vi "Parse Global Header.vi"(8 "error in":errorcluster, 10 "Bytes in":u8[](array[numeric]), 11 "pcap Parse and Build in":refnum<class "pcap_Parse_Build_CIF.lvclass">) -> (0 "error out":errorcluster, 1 "Global Header":T1 {"magic number" format="%.0x"}, 2 "Bytes out":u8[](array[numeric]), 3 "pcap Parse and Build out":refnum<class "pcap_Parse_Build_CIF.lvclass">)   [LabVIEW 2021, in "pcap_Parse_Build_CIF.lvclass"]
uses:
  pcap_Parse_Build_CIF.lvclass
  Typedef/Global Header.ctl
  Typedef/Errors.ctl
  Typedef/Time Format.ctl
  Typedef/File Format.ctl
  <vilib>/CIF Foundation/CIF Utilities/DataTypes/Typedef/Endian.ctl
  pcap_Parse_Build_CIF.lvclass/pcap_Parse_Build_CIF.ctl
  Utilities/Add Error Core.vi
  <vilib>/CIF Foundation/CIF Utilities/DataTypes/DataTypes_CIF_U.lvlib
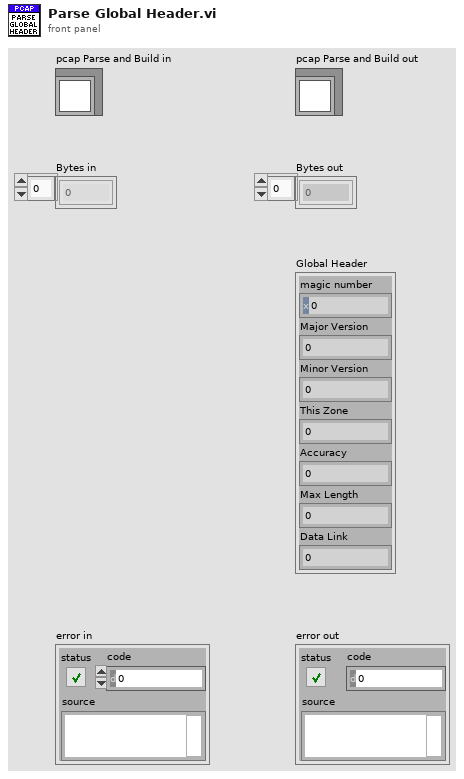
[diagram p1: front panel]
types:
  T1 = typedef "pcap_Parse_Build_CIF.lvclass/Global Header.ctl" = cluster{"magic number":u32, "Major Version":u16, "Minor Version":u16, "This Zone":u32, "Accuracy":u32, "Max Length":u32, "Data Link":u32}
  T2 = typedef "pcap_Parse_Build_CIF.lvclass/Errors.ctl" = enum16{"Invalid Global Header", "Out of Data"}
  T3 = typedef "pcap_Parse_Build_CIF.lvclass/Time Format.ctl" = enum16{"us", "ns"}
  T4 = typedef "pcap_Parse_Build_CIF.lvclass/File Format.ctl" = cluster{"Endian":T5, "Time Format":T3}
  T5 = typedef "DataTypes_CIF_U.lvlib/Endian.ctl" = enum16{"Little Endian", "Big Endian"}
  T6 = enum16{"big-endian, network order", "native, host order", "little-endian"}[]
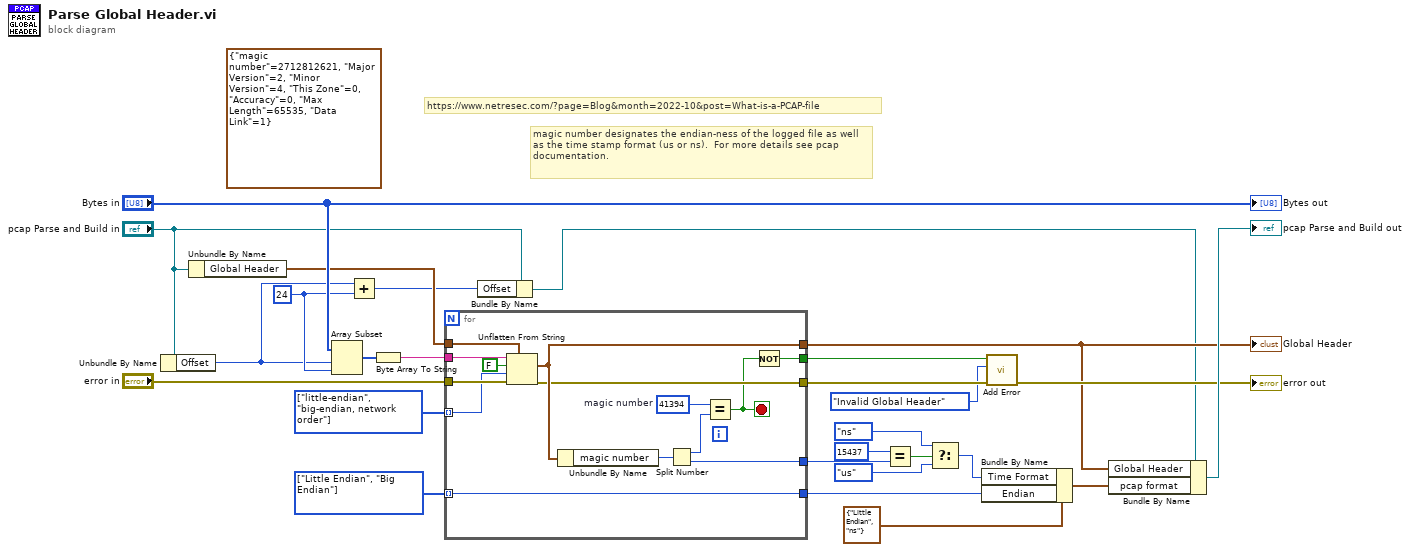
[diagram p0: block diagram]
diagram:
  w16 = T5[] [enum."Little Endian", enum."Big Endian"] items=["Little Endian", "Big Endian"]
  w18 = 24 ("y")
  (unwired) T1 {"magic number"=2712812621, "Major Version"=2, "Minor Version"=4, "This Zone"=0, "Accuracy"=0, "Max Length"=65535, "Data Link"=1} ("Global Header")
  w26 = T6 [enum."little-endian", enum."big-endian, network order"] items=["big-endian, network order", "native, host order", "little-endian"]
  # "https://www.netresec.com/?page=Blog&month=2022-10&post=What-is-a-PCAP-file"
  # "magic number designates the endian-ness of the logged file as well as the time stamp format (us or ns).  For more details see pcap documentation."
  n1 = Unbundle By Name("pcap Parse and Build in") -> ("Offset"=w4:i32)
  n2 = Unbundle By Name("pcap Parse and Build in") -> ("Global Header"=w5:T1)
  n3 = Array Subset(array="Bytes in", index=w4, length=w18) -> (w17:u8[])
  n4 = Add(x=w4, y=w18) -> (x+y=w2:i32)
  n5 = Byte Array To String(unsigned byte array=w17) -> (string=w27:string)
  n6 = for {
    tunnel: w27 -> [w41]
    tunnel: w26 -> [w30] mode=indexing
    tunnel: [w39] -> w6
    tunnel: [w31] -> w21
    tunnel: [w29] -> w8
    tunnel: [w35] -> w25
    tunnel: [w34] -> w10
    tunnel: "error in" -> [w33]
    tunnel: w16 -> [w31] mode=indexing
    tunnel: w5 -> [w28]
    stop <- w32 stop-if-true
    w36 = u16 41394  # magic number
    n7 = Unflatten From String(type=w28, binary string=w41, data includes array or string size? (T)=FALSE, byte order (0:big-endian, network order)=w30, error in (no error)=w33) -> (value=w39:T1, error out=w34:errorcluster)  [unwired: 1 out]
    n8 = Unbundle By Name(w39) -> ("magic number"=w38:u32)
    n9 = Split Number(x=w38) -> (hi(x)=w37:u16, lo(x)=w35:u16)
    n10 = Equal?(x=w36, y=w37) -> (x = y?=w32:bool)
    n11 = Not(x=w32) -> (.not. x?=w29:bool)
  }
  "Global Header" <- w6
  n12 = Bundle By Name(cluster="pcap Parse and Build in", "Offset"=w2) -> (w1:refnum<class "pcap_Parse_Build_CIF.lvclass">)
  n13 = Equal?(x=u16 15437, y=w25) -> (x = y?=w23:bool)
  n14 = Select(t=Time_Format."ns" ("Time Format"), s=w23, f=Time_Format."us" ("Time Format")) -> (s? t:f=w20:T3)
  n15 = Bundle By Name(cluster=T4 {"Endian"=enum."Little Endian", "Time Format"=enum."ns"} ("File Format"), "Time Format"=w20, "Endian"=w21) -> (w12:T4)
  n16 = call "Add Error.vi"("error in (no error)"=w10, "Error"=Errors."Invalid Global Header", "Insert Error"=w8) -> ("error out"=→"error out":errorcluster)  [unwired: 8 in]
  n17 = Bundle By Name(cluster=w1, "Global Header"=w6, "pcap format"=w12) -> (→"pcap Parse and Build out":refnum<class "pcap_Parse_Build_CIF.lvclass">)
  "Bytes out" <- "Bytes in"
